vi "Write Camera.vi"(10 "Camera.lvclass":refnum<class "Camera.lvclass">, 11 "Experiment in":refnum<class "Experiment.lvclass">) -> (3 "Experiment out":refnum<class "Experiment.lvclass">)   [LabVIEW 2013]
uses:
  Experiment.lvclass
  Camera/Camera.lvclass
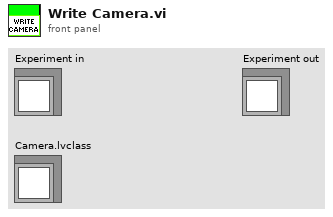
[diagram p1: front panel]
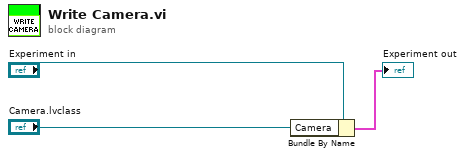
[diagram p0: block diagram]
diagram:
  n1 = Bundle By Name(cluster="Experiment in", "Camera"="Camera.lvclass") -> (→"Experiment out":cluster{})
